vi "External Actuator Daq Send.vi"(8 "error in (no error)":errorcluster, 10 "Commands":dbl[](array[numeric]), 11 "Daq Actions":T1) -> (0 "error out":errorcluster)   [LabVIEW 2009]
uses:
  Daq Actions.ctl
  <vilib>/DAQmx/write.llb/DAQmx Write (Analog 1D DBL NChan 1Samp).vi
panel:
  out "Channels":refnum<k21>
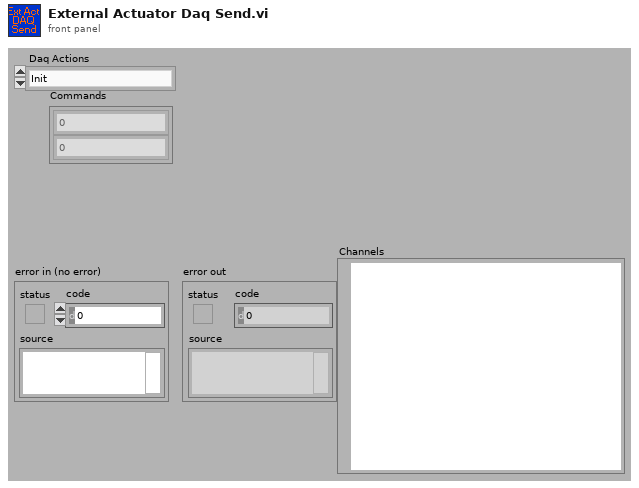
[diagram p1: front panel]
types:
  T1 = typedef "Daq Actions.ctl" = enum16{"Init", "Send Commands", "Get Responses", "Stop"}
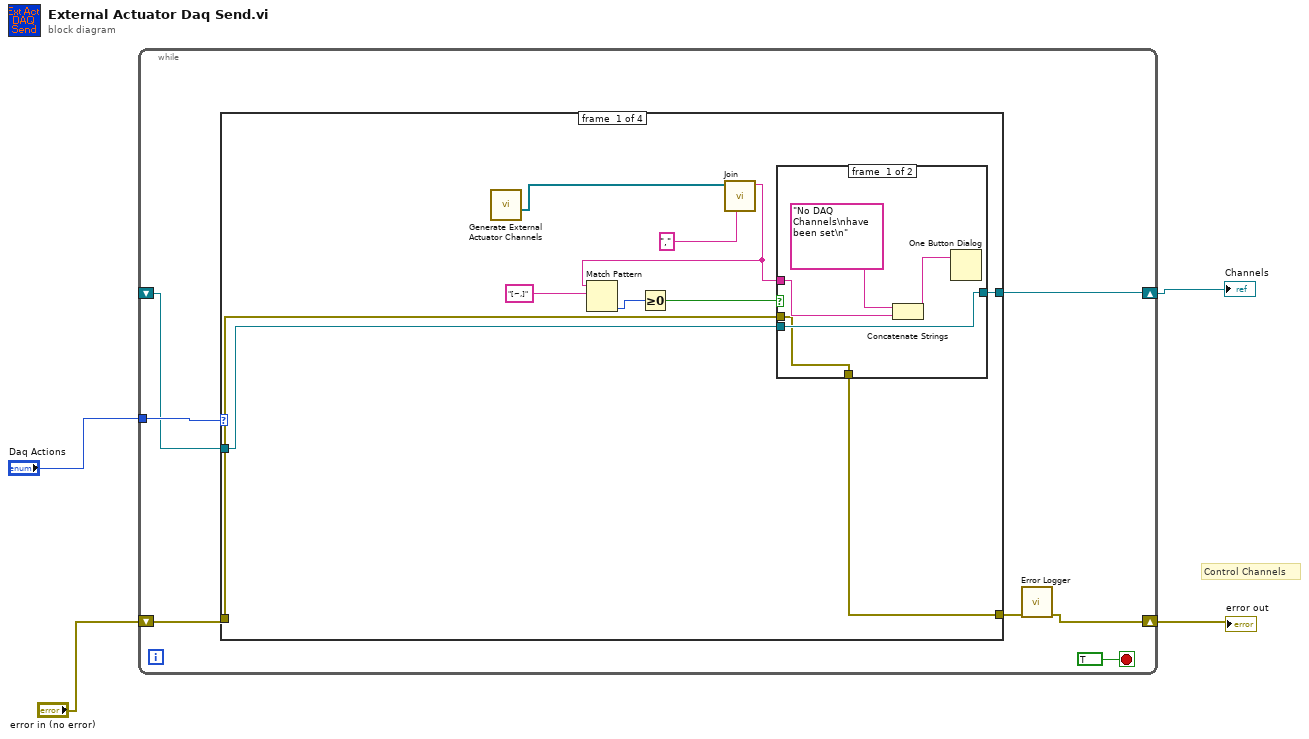
[diagram p0: block diagram]
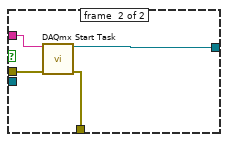
[diagram p2: hidden frame]
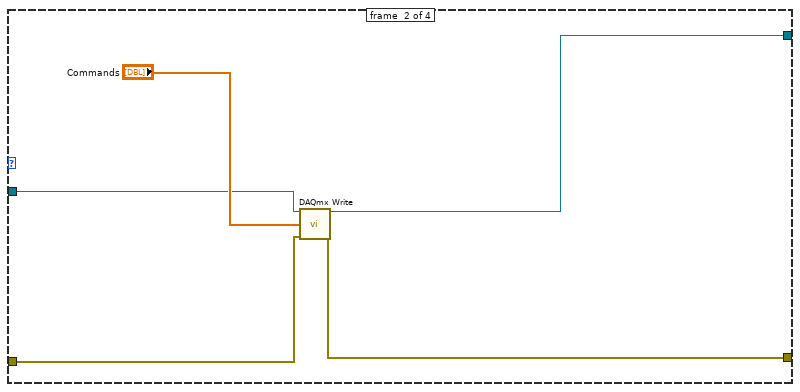
[diagram p3: hidden frame]
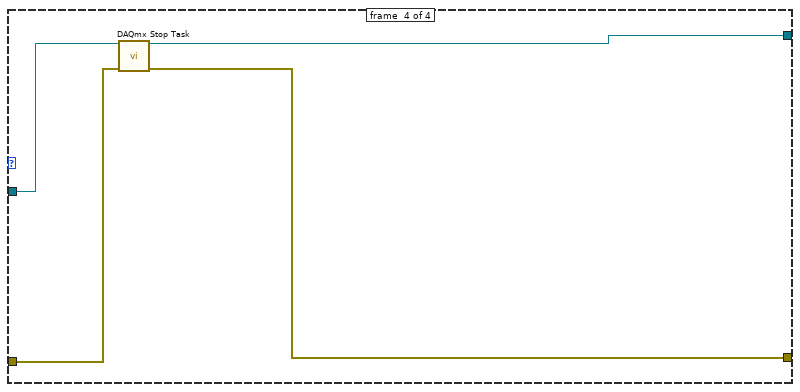
[diagram p5: hidden frame]
diagram:
  # "Control Channels"
  n1 = while {
    tunnel: "Daq Actions" -> [w11]
    shift-right: [w9] -> w1
    shift-left: _ -> [w8]
    shift-right: [w6] -> w2
    shift-left: "error in (no error)" -> [w7]
    stop <- TRUE stop-if-true
    n2 = case shown="\"Send Commands\"" w11 {
      tunnel: [w21 w32 w37 w41] -> w9
      tunnel: w8 -> [w14 w31 w37 w40]
      tunnel: w7 -> [w20 w34 w36 w39]
      tunnel: [w12 w33 w36 w38] -> w5
      frame #0 {
        n3 = call "Generate External Actuator Channels.vi"() -> ("Output Channels"=w13:refnum<k21>[])  [unwired: 10 in, 1 out]
        n4 = call "Join.vi"("delimiter"=",", "Array"=w13) -> ("Joined Result"=w15:string)  [unwired: 9 out]
        n5 = Match Pattern(string=w15, regular expression="[~,]") -> (offset past match=w17:i32)  [unwired: 4 out]
        n6 = Greater Or Equal To 0?(x=w17) -> (x >= 0?=w16:bool)
        n7 = case shown="False" w16 {
          tunnel: [w23 w30] -> w21
          tunnel: w20 -> [w22 w29]
          tunnel: [w22 w28] -> w12
          tunnel: w15 -> [w24 w27]
          tunnel: w14 -> [w23 _]
          frame #0 {
            n8 = Concatenate Strings("No DAQ Channels\nhave been set\n" ("string"), w24) -> (w25:string)
            n9 = One Button Dialog(message=w25) -> ()  [unwired: 2 out]
          }
          frame #1 {
            n10 = call <vilib>:"DAQmx Start Task.vi"("task/channels in"=w27, "error in"=w29) -> ("task out"=w30:refnum<k21>, "error out"=w28:errorcluster)  [unwired: 12 out]
          }
        }
      }
      frame #1 {
        n11 = call-poly <vilib>:"DAQmx Write.vi"("task/channels in"=w31, "data"="Commands", "error in"=w34) -> ("task out"=w32:refnum<k21>, "error out"=w33:errorcluster)  [unwired: 2 in, 9 out]
      }
      frame #2 {
      }
      frame #3 {
        n12 = call <vilib>:"DAQmx Stop Task.vi"("task/channels in"=w40, "error in"=w39) -> ("task out"=w41:refnum<k21>, "error out"=w38:errorcluster)  [unwired: 12 out]
      }
    }
    n13 = call "Error Logger.vi"("error in (no error)"=w5) -> ("error out"=w6:errorcluster)  [unwired: 1 in, 9 out]
  }
  "error out" <- w2
  "Channels" <- w1
